vi "Read Color Cluster.vi"(8 "error in (no error)":errorcluster, 9 "Active Plot":i32, 11 "3D Plot in":refnum<class "3D Plot.lvclass">) -> (0 "error out":errorcluster, 2 "Color Ramp Cluster":T1={"Color Ramp Style"=enum."None", "Color Ramp Array"=[16711934, 393471, 57855, 4390754, 16449346, 16744722, 16711680], "Color Ramp Index"=[45, 91, 133, 175, 219, 255], "Interpolate?"=FALSE, "Logarithm?"=FALSE}, 3 "3D Plot out":refnum<class "3D Plot.lvclass">)   [LabVIEW 2020, in "3D Plot.lvclass"]
uses:
  3D Plot.lvclass
  Color Ramp Cluster.ctl
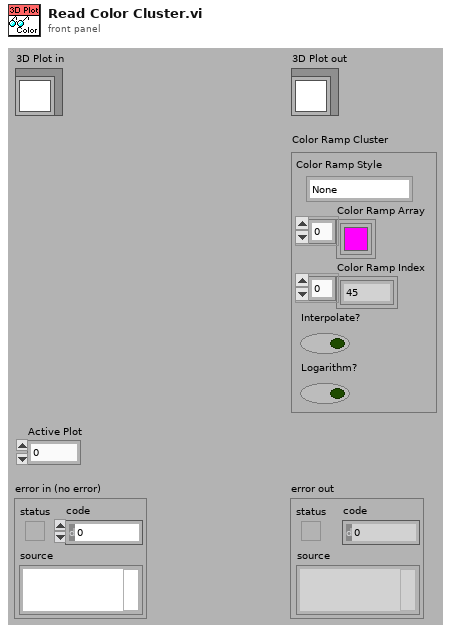
[diagram p1: front panel]
types:
  T1 = typedef "3D Plot.lvclass/Color Ramp Cluster.ctl" = cluster{"Color Ramp Style":enum16{"None", "Shaded", "Color spectrum", "Grey scale", "Custom"}, "Color Ramp Array":u32[], "Color Ramp Index":i32[], "Interpolate?":bool, "Logarithm?":bool}
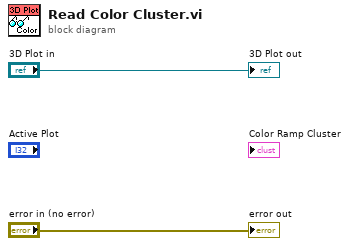
[diagram p0: block diagram]
diagram:
  "error out" <- "error in (no error)"
  "3D Plot out" <- "3D Plot in"
